vi "SmartDashboardInsidePeriodicTasks.vi"() -> ()   [LabVIEW 2012]
panel:
  out "Vertical Angle":dbl
  out "Horizontal Angle":dbl
  out "Distance to center of target":dbl
  in  "visionMode":dbl
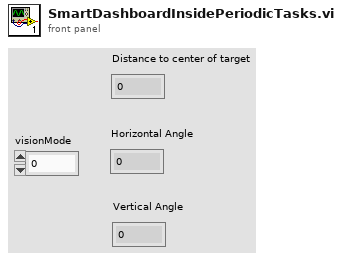
[diagram p1: front panel]
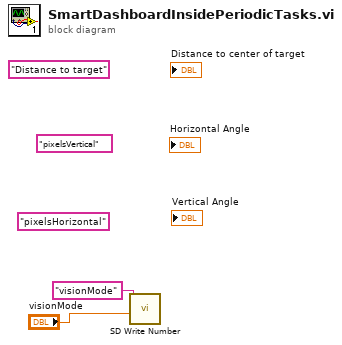
[diagram p0: block diagram]
diagram:
  (unwired) "pixelsHorizontal" ("Name")
  (unwired) "pixelsVertical" ("Name")
  (unwired) "Distance to target" ("Name")
  n1 = call <vilib>:"SD Write Number.vi"("Numeric"="visionMode", "Name"="visionMode") -> ()  [unwired: 8 in, 2 out]
